vi "Parse MISSION_ITEM.vi"(11 "Data":string) -> (3 "Mission Item":T1={"target_system"=0, "target_component"=0, "sequence"=0, "frame"=enum."GLOBAL RELATIVE ALT", "command"=0, "current"=FALSE, "autocontinue"=FALSE, "param1"=0.0, "param2"=0.0, "param3"=0.0, "param4"=0.0, "Lat"=0.0, "Lon"=0.0, "Altitude (m)"=0.0})   [LabVIEW 2014]
uses:
  Controls/Mission Planning Controls/MAVLINK Mission Item.ctl
  Controls/MAVLINK Mav Frame.ctl
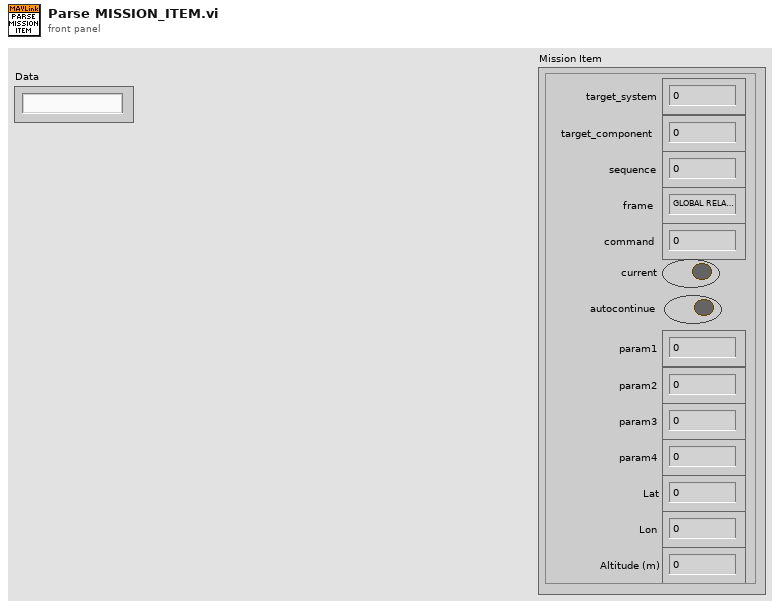
[diagram p1: front panel]
types:
  T1 = typedef "MAVLINK Mission Item.ctl" = cluster{"target_system":u8, "target_component":u8, "sequence":u16, "frame":T2, "command":u16, "current":bool, "autocontinue":bool, "param1":sgl, "param2":sgl, "param3":sgl, "param4":sgl, "Lat":sgl, "Lon":sgl, "Altitude (m)":sgl}
  T2 = typedef "MAVLINK Mav Frame.ctl" = enum8{"GLOBAL", "LOCAL NED", "MISSION", "GLOBAL RELATIVE ALT", "LOCAL ENU", "GLOBAL INT", "GLOBAL RELATIVE ALT INT", "LOCAL OFFSET NED", "BODY NED", "BODY OFFSET NED", "GLOBAL TERRAIN ALT", "GLOBAL TERRAIN ALT INT"}
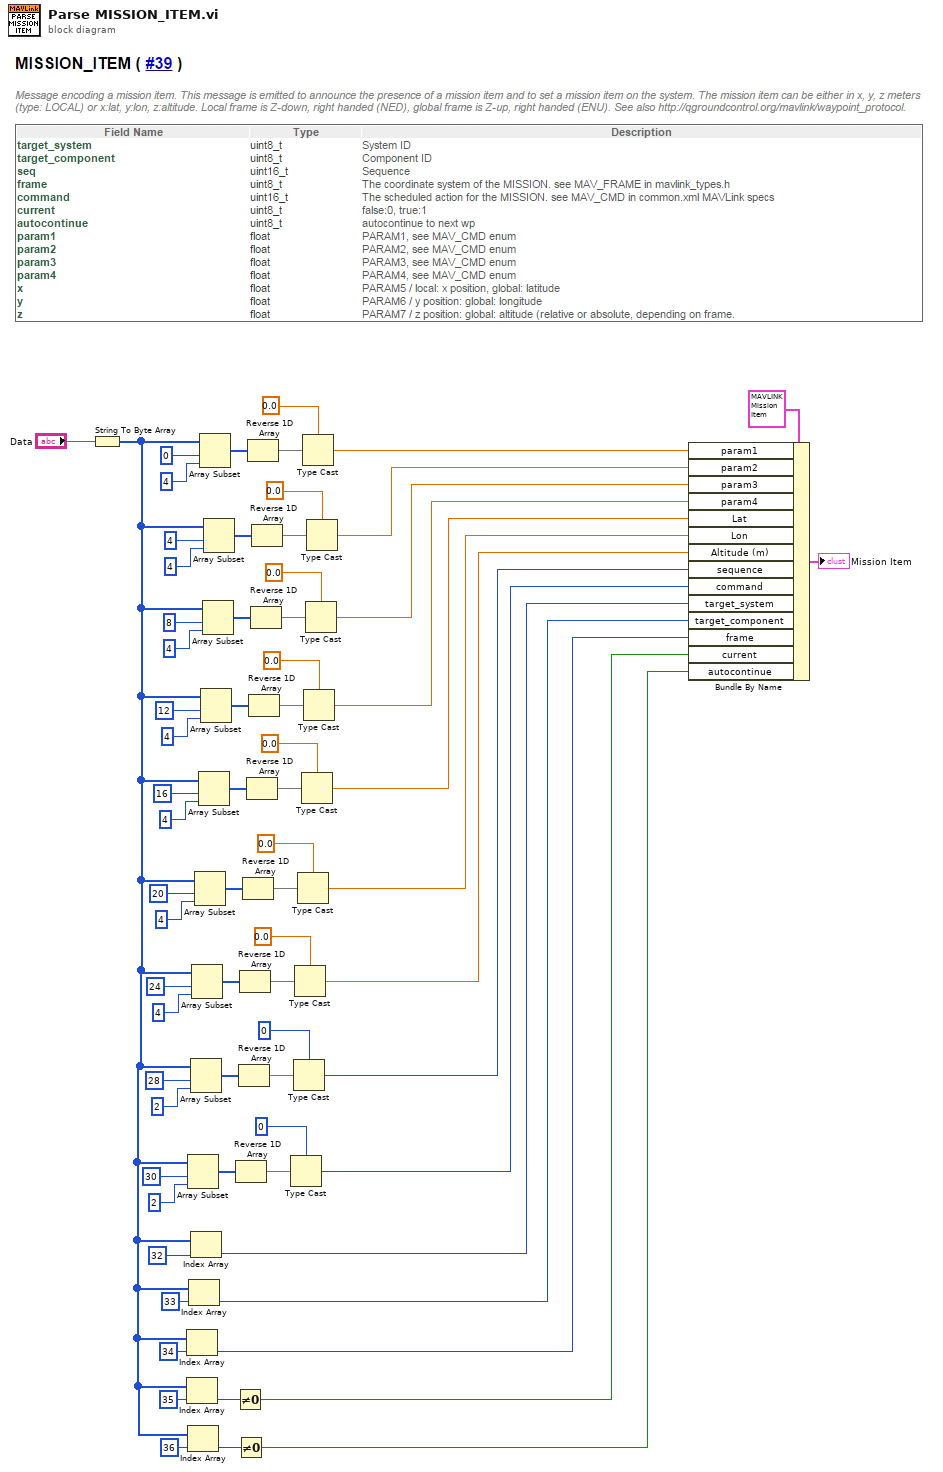
[diagram p0: block diagram]
diagram:
  n1 = String To Byte Array(string="Data") -> (unsigned byte array=w3:u8[])
  n2 = Index Array(array=w3, index=34) -> (element=w9:u8)
  n3 = Index Array(array=w3, index=35) -> (element=w7:u8)
  n4 = Array Subset(array=w3, index=30, length=2) -> (w17:u8[])
  n5 = Index Array(array=w3, index=36) -> (element=w5:u8)
  n6 = Index Array(array=w3, index=33) -> (element=w11:u8)
  n7 = Array Subset(array=w3, index=28, length=2) -> (w25:u8[])
  n8 = Index Array(array=w3, index=32) -> (element=w13:u8)
  n9 = Array Subset(array=w3, index=24, length=4) -> (w29:u8[])
  n10 = Array Subset(array=w3, index=20, length=4) -> (w37:u8[])
  n11 = Array Subset(array=w3, index=16, length=4) -> (w47:u8[])
  n12 = Array Subset(array=w3, index=0, length=4) -> (w68:u8[])
  n13 = Array Subset(array=w3, index=12, length=4) -> (w52:u8[])
  n14 = Array Subset(array=w3, index=8, length=4) -> (w57:u8[])
  n15 = Array Subset(array=w3, index=4, length=4) -> (w61:u8[])
  n16 = Not Equal To 0?(x=w7) -> (x != 0?=w6:bool)
  n17 = Reverse 1D Array(array=w17) -> (reversed array=w16:u8[])
  n18 = Not Equal To 0?(x=w5) -> (x != 0?=w2:bool)
  n19 = Reverse 1D Array(array=w25) -> (reversed array=w26:u8[])
  n20 = Reverse 1D Array(array=w29) -> (reversed array=w28:u8[])
  n21 = Reverse 1D Array(array=w37) -> (reversed array=w38:u8[])
  n22 = Reverse 1D Array(array=w47) -> (reversed array=w46:u8[])
  n23 = Reverse 1D Array(array=w68) -> (reversed array=w69:u8[])
  n24 = Reverse 1D Array(array=w52) -> (reversed array=w51:u8[])
  n25 = Reverse 1D Array(array=w57) -> (reversed array=w56:u8[])
  n26 = Reverse 1D Array(array=w61) -> (reversed array=w60:u8[])
  n27 = Type Cast(type=u16 0 ("single precision float"), x=w16) -> (*(type *) &x=w15:u16)
  n28 = Type Cast(type=u16 0 ("single precision float"), x=w26) -> (*(type *) &x=w21:u16)
  n29 = Type Cast(type=sgl 0.0 ("single precision float"), x=w28) -> (*(type *) &x=w27:sgl)
  n30 = Type Cast(type=sgl 0.0 ("single precision float"), x=w38) -> (*(type *) &x=w33:sgl)
  n31 = Type Cast(type=sgl 0.0 ("single precision float"), x=w46) -> (*(type *) &x=w39:sgl)
  n32 = Type Cast(type=sgl 0.0 ("single precision float"), x=w69) -> (*(type *) &x=w43:sgl)
  n33 = Type Cast(type=sgl 0.0 ("single precision float"), x=w51) -> (*(type *) &x=w40:sgl)
  n34 = Type Cast(type=sgl 0.0 ("single precision float"), x=w56) -> (*(type *) &x=w41:sgl)
  n35 = Type Cast(type=sgl 0.0 ("single precision float"), x=w60) -> (*(type *) &x=w42:sgl)
  n36 = Bundle By Name(cluster=T1 {"target_system"=0, "target_component"=0, "sequence"=0, "frame"=enum."GLOBAL RELATIVE ALT", "command"=0, "current"=FALSE, "autocontinue"=FALSE, "param1"=0.0, "param2"=0.0, "param3"=0.0, "param4"=0.0, "Lat"=0.0, "Lon"=0.0, "Altitude (m)"=0.0} ("MISSION_ITEM"), "param1"=w43, "param2"=w42, "param3"=w41, "param4"=w40, "Lat"=w39, "Lon"=w33, "Altitude (m)"=w27, "sequence"=w21, "command"=w15, "target_system"=w13, "target_component"=w11, "frame"=w9, "current"=w6, "autocontinue"=w2) -> (→"Mission Item":T1)
